vi "EDIT ITEMS IN PGSQL.vi"(11 "DATA IN":T1[](array[typedef])) -> ()   [LabVIEW 2019]
uses:
  Controls/Table Data Types/Inventory Data Type.ctl
  Controls/Column Names/Inventory Column Names.ctl
  <vilib>/addons/database/Connection.llb/DB Tools Open Connec (String).vi
  <vilib>/addons/database/NI_Database_API.lvlib
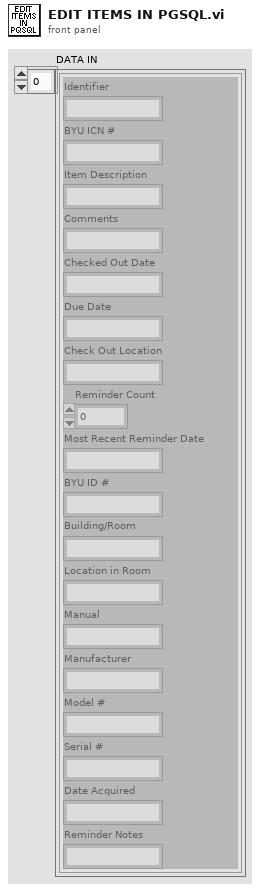
[diagram p1: front panel]
types:
  T1 = typedef "Inventory Data Type.ctl" = cluster{"Identifier":string, "BYU ICN #":string, "Item Description":string, "Comments":string, "Checked Out Date":string, "Due Date":string, "Check Out Location":string, "Reminder Count":i32, "Most Recent Reminder Date":string, "BYU ID #":string, "Building/Room":string, "Location in Room":string, "Manual":string, "Manufacturer":string, "Model #":string, "Serial #":string, "Date Acquired":string, "Reminder Notes":string}
  T2 = typedef "NI_Database_API.lvlib/Conn ObjectReference.ctl" = refnum<k1>
  T3 = typedef "Inventory Column Names.ctl" = string[]
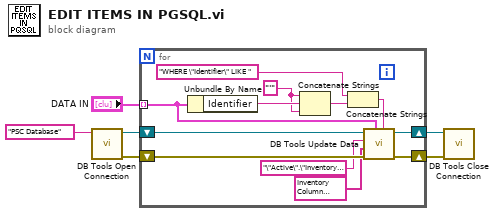
[diagram p0: block diagram]
diagram:
  n1 = call-poly <vilib>:"DB Tools Open Connection.vi"("connection information"="PSC Database" ("string")) -> ("error out"=w5:errorcluster, "connection reference"=w6:T2)  [unwired: 7 in]
  n2 = for {
    shift-right: [w12] -> w3
    shift-left: w6 -> [w18]
    shift-right: [w11] -> w2
    shift-left: w5 -> [w17]
    tunnel: "DATA IN" -> [w14] mode=indexing
    w8 = "'" ("string")
    n3 = Unbundle By Name(w14) -> ("Identifier"=w9:string)
    n4 = Concatenate Strings(w8, w9, w8) -> (w10:string)
    n5 = Concatenate Strings("WHERE \"Identifier\" LIKE " ("string"), w10) -> (w15:string)
    n6 = call <vilib>:"DB Tools Update Data.vi"("condition"=w15, "data"=w14, "error in (no error)"=w17, "columns"=T3 ["\"Identifier\"", "\"BYU ICN #\"", "\"Item Description\"", "\"Comments\"", "\"Checked Out Date\"", "\"Due Date\"", "\"Check Out Location\"", "\"Reminder Count\"", "\"Most Recent Reminder Date\"", "\"BYU ID #\"", "\"Building/Room\"", "\"Location in Room\"", "\"Manual\"", "\"Manufacturer\"", "\"Model #\"", "\"Serial #\"", "\"Date Acquired\""] ("INVENTORY COLUMN NAMES"), "table"="\"Active\".\"Inventory\"" ("string"), "connection reference"=w18) -> ("error out"=w11:errorcluster, "connection reference out"=w12:T2)  [unwired: 4 in]
  }
  n7 = call <vilib>:"DB Tools Close Connection.vi"("error in (no error)"=w2, "connection reference"=w3) -> ()  [unwired: 5 in, 1 out]
